vi "SSL Detection Frame Robots Estimator.vi"(5 "Time Stamp":timestamp, 7 "Life Time":dbl=1.0, 11 "Robots":T1[](array[typedef]) {"height" format="%+4.3f"; "pixel_y" format="%+4.3f"; "pixel_x" format="%+4.3f"; "orientation" format="%+4.3f"; "y" format="%+4.3f"; "confidence" format="%4.3f"; "x" format="%+4.3f"}) -> (3 "Est. Robots":T1[](array[typedef]) {"height" format="%+4.3f"; "pixel_y" format="%+4.3f"; "pixel_x" format="%+4.3f"; "orientation" format="%+4.3f"; "y" format="%+4.3f"; "confidence" format="%4.3f"; "x" format="%+4.3f"})   [LabVIEW 2016]
uses:
  SSL Detection Robot.ctl
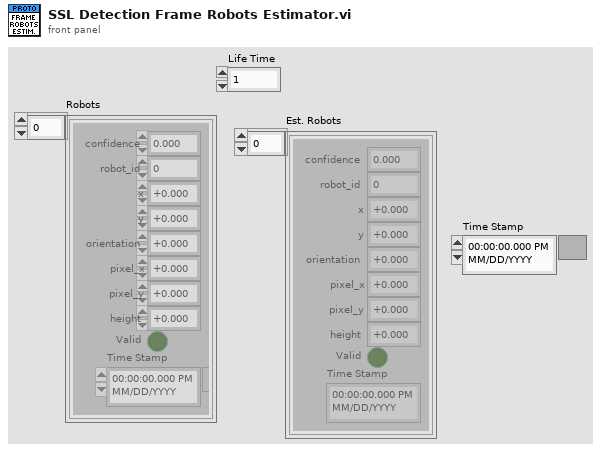
[diagram p1: front panel]
types:
  T1 = typedef "SSL Detection Robot.ctl" = cluster{"x":dbl, "robot_id":u32, "confidence":sgl, "y":sgl, "orientation":sgl, "pixel_x":sgl, "pixel_y":sgl, "height":sgl, "Valid":bool, "Time Stamp":timestamp}
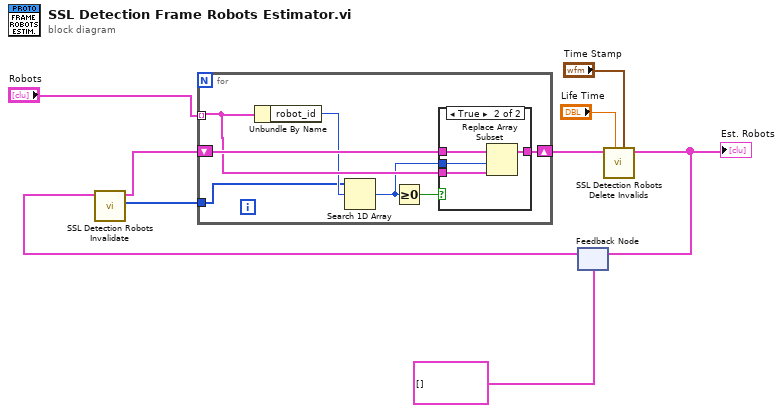
[diagram p0: block diagram]
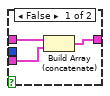
[diagram p2: hidden frame]
diagram:
  n1 = feedback #1(T1[] [] ("Robots Out")) -> (w2:T1[])
  n2 = call "SSL Detection Robots Invalidate.vi"("Robots"=w2) -> ("Indexes"=w4:u32[], "Robots Invalidated"=w6:T1[])  [unwired: 9 in]
  n3 = for {
    tunnel: "Robots" -> [w14] mode=indexing
    shift-right: [w15] -> w5
    shift-left: w6 -> [w16]
    tunnel: w4 -> [w12]
    n4 = Unbundle By Name(w14) -> ("robot_id"=w13:u32)
    n5 = Search 1D Array(1D array=w12, element=w13) -> (index of element=w10:i32)  [unwired: 1 in]
    n6 = Greater Or Equal To 0?(x=w10) -> (x >= 0?=w11:bool)
    n7 = case shown="True" w11 {
      tunnel: w16 -> [w18 w23]
      tunnel: [w17 w22] -> w15
      tunnel: w14 -> [w19 w21]
      tunnel: w10 -> [_ w20]
      frame False {
        n8 = Build Array (concatenate)(w18, w19) -> (w17:T1[])
      }
      frame True {
        n9 = Replace Array Subset(array=w23, new element=w21, index=w20) -> (w22:T1[])
      }
    }
  }
  n10 = call "SSL Detection Robots Delete Invalids.vi"("Now"="Time Stamp", "Life Time"="Life Time", "Robots In"=w5) -> ("Robots Out"=w3:T1[])  [unwired: 8 in]
  "Est. Robots" <- w3
  n11 = feedback-in #1(w3) -> ()
